vi "sonarSetLights.vi"(0 "error in":errorcluster, 2 "Lights":T1, 3 "node":string) -> (1 "error out":errorcluster)   [LabVIEW 2010]
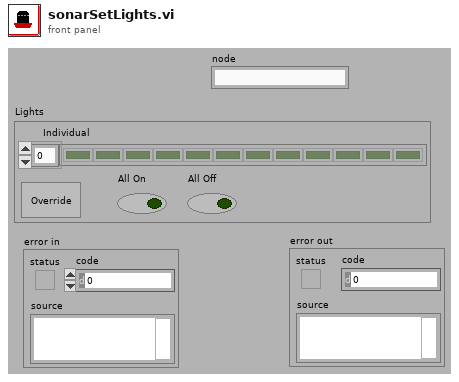
[diagram p1: front panel]
types:
  T1 = cluster{"Behavior":bool, "All On":bool, "All Off":bool, "Individual":bool[]}
  T2 = typedef "_ROSControl.ctl" = cluster{"topic port":u16, "Node":string, "topic":string, "type":string, "node port":u32, "error ":errorcluster, "Direction":T3, "APIs":string[]}
  T3 = typedef "_ROSDirection.ctl" = enum16{"Node", "Publisher", "Subscriber", "Service Client"}
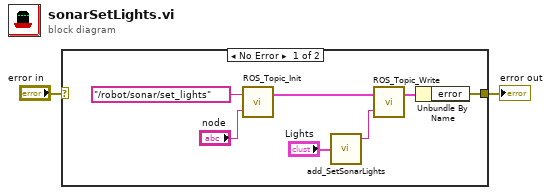
[diagram p0: block diagram]
diagram:
  n1 = case shown="No Error" "error in" {
    selector: "error in" -> [_ w10]
    tunnel: [w9 w10] -> w2
    frame No Error {
      n2 = call <userlib>:"ROS_Topic_Init.vi"("node"="node", "topic"="/robot/sonar/set_lights") -> ("ROS out"=w6:T2)  [unwired: 1 in]
      n3 = call <userlib>:"add_SetSonarLights.vi"("Lights"="Lights") -> ("msg out"=w3:string)  [unwired: 4 in]
      n4 = call <userlib>:"ROS_Topic_Write.vi"("Msg in"=w3, "ROS in"=w6) -> ("ROS out"=w5:T2)  [unwired: 1 in]
      n5 = Unbundle By Name(w5) -> ("error"=w9:errorcluster)
    }
    frame Error {
    }
  }
  "error out" <- w2
